vi "UpdateIO.vi"(11 "Count(ticks)":u32=20) -> ()   [LabVIEW 2009]
uses:
  <vilib>/eio/EIONode/EIONode.xnode
  <vilib>/rvi/eio/nirviEIOImplementation/nirviEIOImplementation.xnode
  <vilib>/rvi/eio/common/nirviEmuTemplateMethod_noerrors.vi
  <vilib>/rvi/eio/common/nirviEmuClasses.ctl
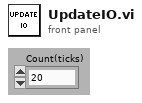
[diagram p1: front panel]
types:
  T1 = typedef "nirviEmuClasses.ctl" = enum16{"IO Read", "IO Write", "Method", "Property Read", "Property Write"}
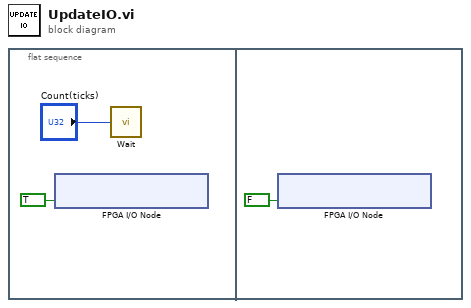
[diagram p0: block diagram]
diagram:
  n1 = flat-sequence {
    frame #0 {
      n2 = xnode "FPGA I/O Node"("IO Module\\UPDATE_IO"=TRUE ("IO Module\\UPDATE_IO")) -> ()  [unwired: 1 in, 1 out]
      n3 = call "Wait"("Count(Ticks)"="Count(ticks)") -> ()  [unwired: 1 out]
    }
    frame #1 {
      n4 = xnode "FPGA I/O Node"("IO Module\\UPDATE_IO"=FALSE ("IO Module\\UPDATE_IO")) -> ()  [unwired: 1 in, 1 out]
    }
  }
